vi "cook.vi"(8 "error in (no error)":errorcluster, 11 "Toast in":refnum<class "Toast.lvclass">) -> (0 "error out":errorcluster, 3 "Toast out":refnum<class "Toast.lvclass">)   [LabVIEW 2011, in "CookBehaviors.lvlib" / "Toast.lvclass"]
uses:
  Toast.lvclass
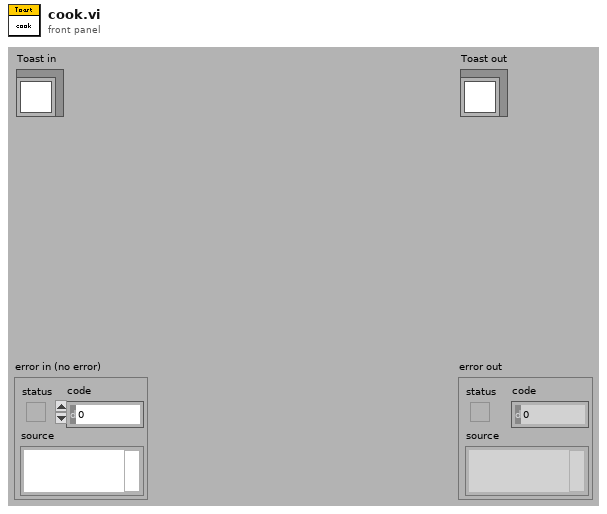
[diagram p1: front panel]
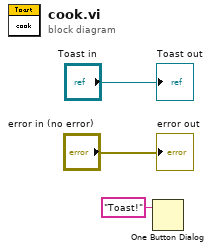
[diagram p0: block diagram]
diagram:
  n1 = One Button Dialog(message="Toast!") -> ()  [unwired: 1 in, 1 out]
  "error out" <- "error in (no error)"
  "Toast out" <- "Toast in"
